vi "Read Requests.vi"(8 "error in (no error)":errorcluster, 11 "TesterModule in":refnum<class "TesterModule.lvclass">) -> (0 "error out":errorcluster, 2 "Requests":T1, 3 "TesterModule out":refnum<class "TesterModule.lvclass">)   [LabVIEW 2024, in "TesterModule.lvclass"]
uses:
  TesterModule.lvclass
  TesterModule.lvclass/TesterModule.ctl
  NewControl78732508.ctl
  NewControl84954098.ctl
  NewControl85010335.ctl
  NewControl85020366.ctl
  NewControl85061316.ctl
  NewControl85443091.ctl
  NewControl85551180.ctl
  NewControl85575480.ctl
  NewControl85623374.ctl
  NewControl85687191.ctl
  NewControl85704585.ctl
  NewControl86016668.ctl
  NewControl86206749.ctl
  NewControl86233597.ctl
  NewControl86273084.ctl
  NewControl86394895.ctl
  NewControl86634965.ctl
  NewControl87012638.ctl
  NewControl87042089.ctl
  NewControl87068529.ctl
  NewControl87087137.ctl
  NewControl87221998.ctl
  NewControl87250161.ctl
  Request Events--cluster.ctl
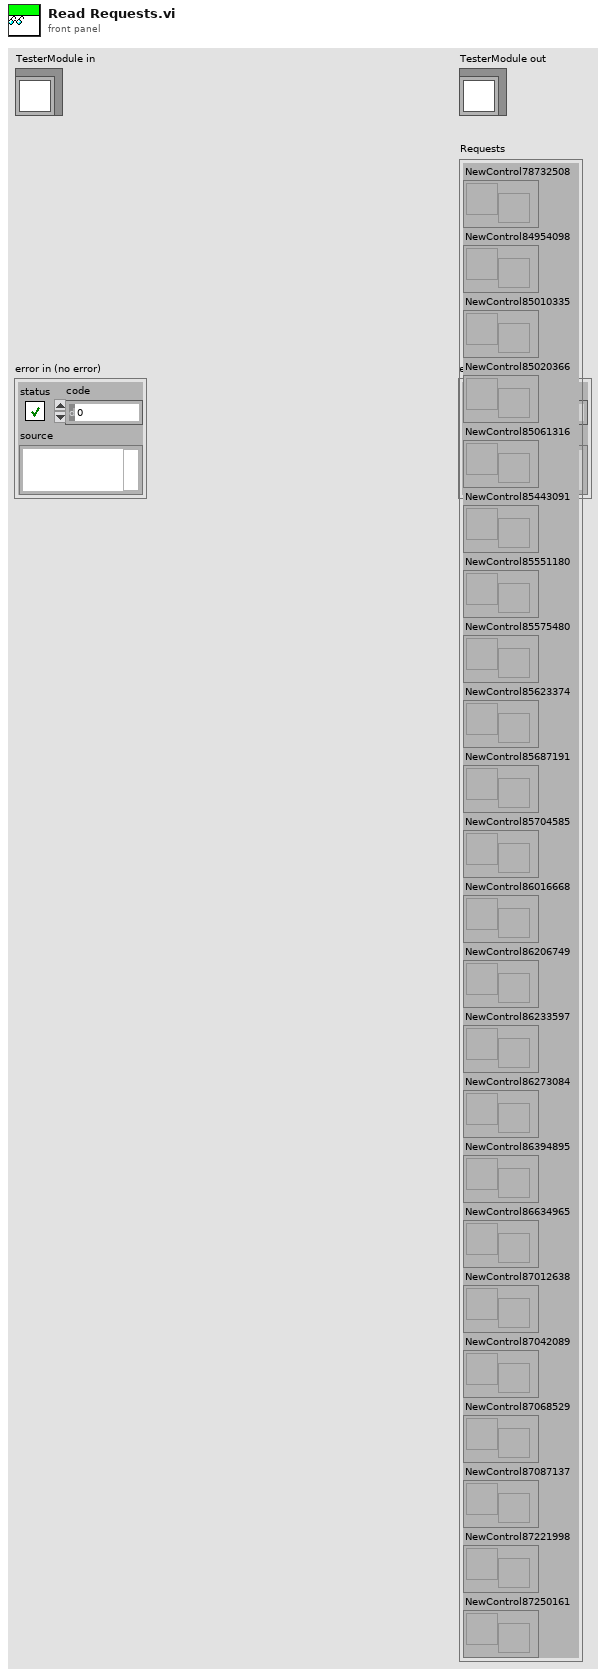
[diagram p1: front panel]
types:
  T1 = typedef "TesterModule.lvclass/Request Events--cluster.ctl" = cluster{"NewControl78732508":refnum<user-event>, "NewControl84954098":refnum<user-event>, "NewControl85010335":refnum<user-event>, "NewControl85020366":refnum<user-event>, "NewControl85061316":refnum<user-event>, "NewControl85443091":refnum<user-event>, "NewControl85551180":refnum<user-event>, "NewControl85575480":refnum<user-event>, "NewControl85623374":refnum<user-event>, "NewControl85687191":refnum<user-event>, "NewControl85704585":refnum<user-event>, "NewControl86016668":refnum<user-event>, "NewControl86206749":refnum<user-event>, "NewControl86233597":refnum<user-event>, "NewControl86273084":refnum<user-event>, "NewControl86394895":refnum<user-event>, "NewControl86634965":refnum<user-event>, "NewControl87012638":refnum<user-event>, "NewControl87042089":refnum<user-event>, "NewControl87068529":refnum<user-event>, "NewControl87087137":refnum<user-event>, "NewControl87221998":refnum<user-event>, "NewControl87250161":refnum<user-event>}
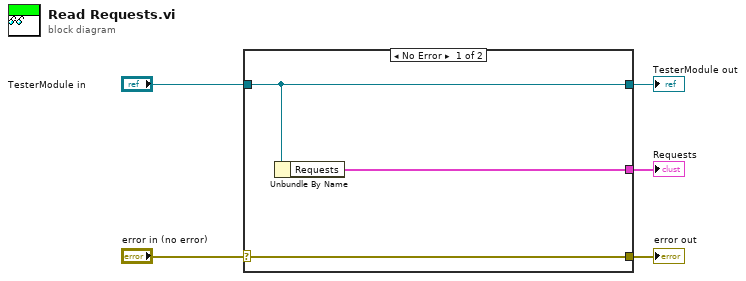
[diagram p0: block diagram]
diagram:
  n1 = case shown="No Error" "error in (no error)" {
    selector: "error in (no error)" -> [w8 w9]
    tunnel: [w8 w9] -> w4
    tunnel: [w7 w10] -> w2
    tunnel: "TesterModule in" -> [w7 w10]
    tunnel: [w6 _] -> w1
    frame No Error {
      n2 = Unbundle By Name(w7) -> ("Requests"=w6:T1)
    }
    frame Error {
    }
  }
  "error out" <- w4
  "TesterModule out" <- w2
  "Requests" <- w1
